vi "Enqueue Close API.vi"(8 "Error In":errorcluster, 11 "Name":string) -> (0 "Error Out":errorcluster)   [LabVIEW 2019, in "FX5U SLMP Binary.lvlib"]
uses:
  FX5U SLMP Binary.lvlib
  Queue/Queue.lvlib
  Error Notifier/Error Notifier.lvlib
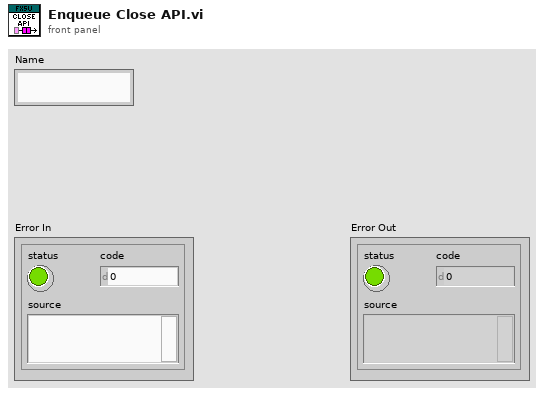
[diagram p1: front panel]
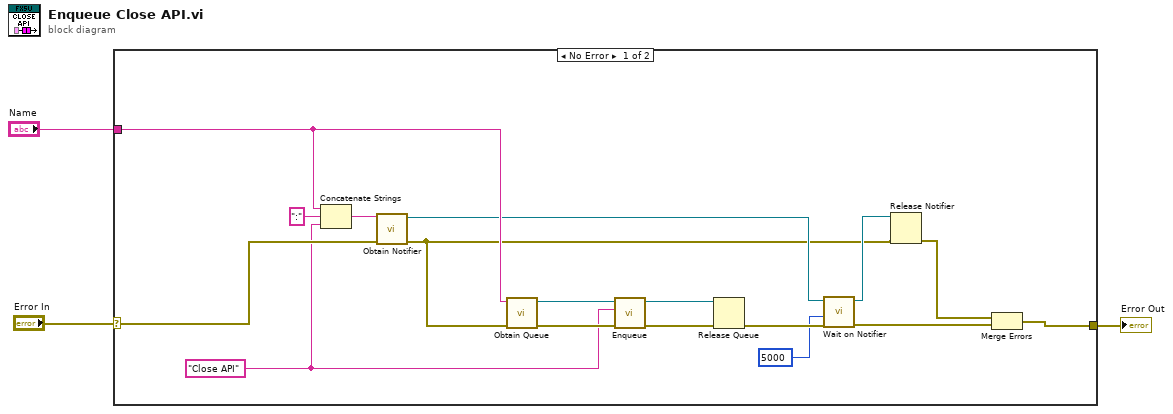
[diagram p0: block diagram]
diagram:
  n1 = case shown="No Error" "Error In" {
    selector: "Error In" -> [w20 w21]
    tunnel: [w5 w21] -> w2
    tunnel: "Name" -> [w18 _]
    frame No Error {
      w15 = "Close API" ("Message")
      n2 = Concatenate Strings(w18, ":" ("string"), w15) -> (w17:string)
      n3 = call "Obtain Notifier.vi"("Error In"=w20, "Name"=w17) -> ("Error Out"=w4:errorcluster, "notifier out"=w10:refnum<notifier>)  [unwired: 8 in]
      n4 = call "Obtain Queue.vi"("Error In"=w4, "Name"=w18) -> ("Error Out"=w19:errorcluster, "queue out"=w13:refnum<queue>)  [unwired: 8 in]
      n5 = call "Enqueue.vi"("Error In"=w19, "Message"=w15, "queue in"=w13) -> ("Error Out"=w14:errorcluster, "queue out"=w12:refnum<queue>)  [unwired: 7 in]
      n6 = Release Queue(queue=w12, error in (no error)=w14) -> (error out=w11:errorcluster)  [unwired: 1 in, 2 out]
      n7 = call "Wait on Notifier.vi"("Error In"=w11, "timeout in ms (-1)"=5000, "notifier in"=w10) -> ("Error Out"=w6:errorcluster, "notifier out"=w8:refnum<notifier>)  [unwired: 7 in]
      n8 = Release Notifier(notifier=w8, error in (no error)=w4) -> (error out=w7:errorcluster)  [unwired: 1 in, 2 out]
      n9 = Merge Errors(w7, w6) -> (w5:errorcluster)
    }
    frame Error {
    }
  }
  "Error Out" <- w2
